vi "Host Main.vi"() -> ()   [LabVIEW 2015]
doc: "This application launches and executes the Tag Bus Data framework configuration for the specified target alias. This is a simple example of the framework API functions, but may also be a suitable starting point for a Host UI or Thick Client that is running a local version of the framework."
uses:
  <vilib>/NI/Module Execution Interface/Engine Runtime/Execution States.ctl
  <vilib>/NI/Module Execution Interface/Engine Runtime/Fault.ctl
  <vilib>/NI/Tag Bus Module Framework/runtime/error classification.ctl
  <vilib>/NI/Module Execution Interface/Engine Runtime/Engine Runtime Interface.lvclass
  <vilib>/NI/DCAF/Tag Editor Core/Framework Configuration Classes/target runtime/PL_Target Runtime.lvclass
  <vilib>/NI/Tag Bus Module Framework/runtime/TBM module execution interface.lvclass
panel:
  in  "configuration file path":path
  in  "target alias":string="PC"
  out "engine status":T4(array[cluster])
  in  "stop":bool
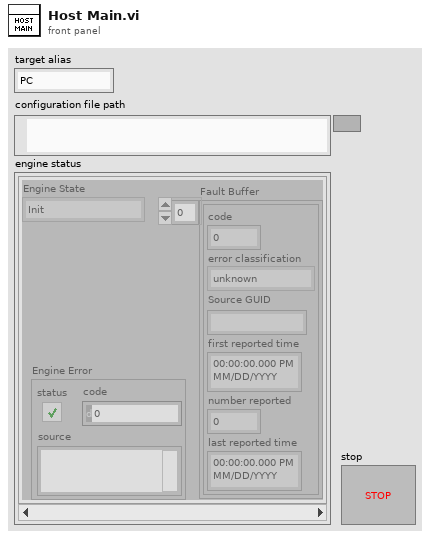
[diagram p1: front panel]
types:
  T1 = typedef "Engine Runtime Interface.lvclass/Execution States.ctl" = enum16{"Init", "Pre-Operational", "Safe-Operational", "Operational", "Stopped"}
  T2 = typedef "Engine Runtime Interface.lvclass/Fault.ctl" = cluster{"code":i32, "error classification":T3, "Source GUID":string, "first reported time":timestamp, "number reported":u32, "last reported time":timestamp}
  T3 = typedef "TBM module execution interface.lvclass/error classification.ctl" = enum16{"unknown", "none", "trivial", "recoverable", "critical"}
  T4 = cluster{"Engine State":T1, "Fault Buffer":T2[], "Engine Error":errorcluster}[]
  T5 = cluster{"Engine State":T1, "Fault Buffer":T2[], "Engine Error":errorcluster}
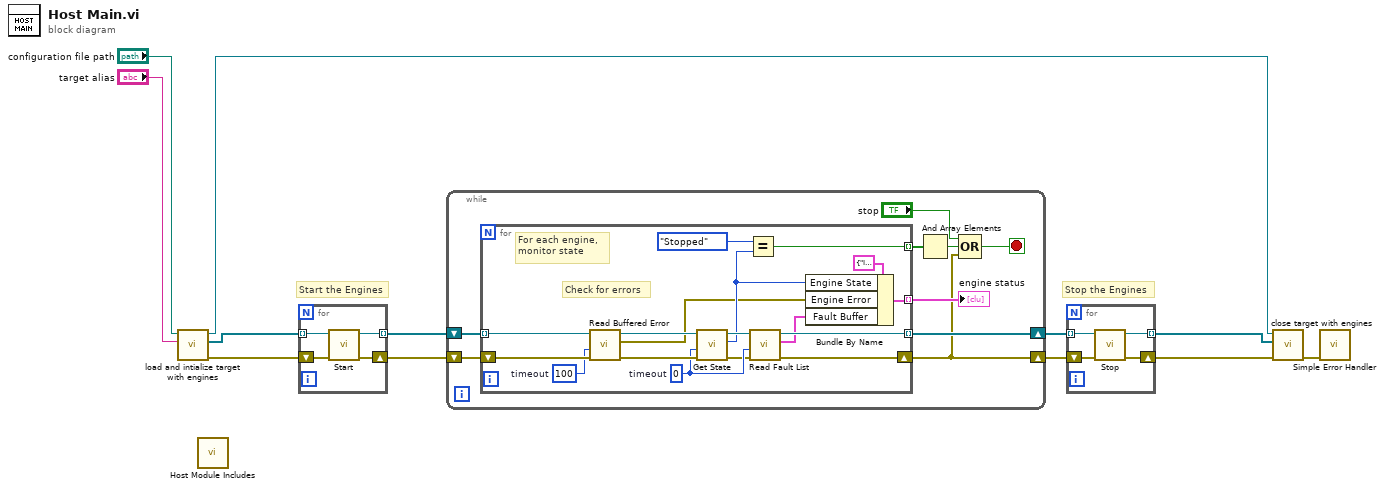
[diagram p0: block diagram]
diagram:
  # "Start the Engines"
  # "Stop the Engines"
  n1 = call <vilib>:"load and intialize target with engines.vi"("target alias"="target alias", "file path"="configuration file path") -> ("error out"=w9:errorcluster, "engine runtime interfaces"=w8:refnum<class "Engine Runtime Interface.lvclass">[], "target runtime"=w5:refnum<class "PL_Target Runtime.lvclass">)  [unwired: 7 in]
  n2 = call "Host Module Includes.vi"() -> ()  [unwired: 12 in]
  n3 = for {
    tunnel: [w16] -> w12 mode=indexing
    tunnel: w8 -> [w13] mode=indexing
    shift-right: [w15] -> w2
    shift-left: w9 -> [w14]
    n4 = call-dynamic "Start.vi"("error in"=w14, "Engine Runtime Interface in"=w13) -> ("error out"=w15:errorcluster, "Engine Runtime Interface out"=w16:refnum<class "Engine Runtime Interface.lvclass">)  [unwired: 8 in]
  }
  n5 = while {
    shift-right: [w23] -> w11
    shift-left: w12 -> [w25]
    shift-right: [w17] -> w10
    shift-left: w2 -> [w24]
    stop <- w21 stop-if-true
    n6 = for {
      tunnel: w25 -> [w42] mode=indexing
      tunnel: [w34] -> w23 mode=indexing
      tunnel: [w37] -> w19 mode=indexing
      shift-right: [w33] -> w17
      shift-left: w24 -> [w41]
      tunnel: [w29] -> w20 mode=indexing
      w32 = 0  # timeout
      w36 = 100  # timeout
      # "For each engine, \nmonitor state"
      # "Check for errors"
      n7 = call-dynamic "Read Buffered Error.vi"("error in"=w41, "timeout in ms (0)"=w36, "Engine Runtime Interface in"=w42) -> ("error out"=w39:errorcluster, "Engine Error"=w27:errorcluster, "Engine Runtime Interface out"=w40:refnum<class "Engine Runtime Interface.lvclass">)  [unwired: 6 in]
      n8 = call-dynamic "Get State.vi"("error in"=w39, "timeout (-1)"=w32, "Engine Runtime Interface in"=w40) -> ("error out"=w26:errorcluster, "Engine State"=w31:T1, "Engine Runtime Interface out"=w35:refnum<class "Engine Runtime Interface.lvclass">)  [unwired: 6 in]
      n9 = Equal?(x=Execution_States."Stopped" ("Engine State"), y=w31) -> (x = y?=w37:bool)
      n10 = call-dynamic "Read Fault List.vi"("error in"=w26, "timeout (-1)"=w32, "Engine Runtime Interface in"=w35) -> ("error out"=w33:errorcluster, "faults"=w30:T2[], "Engine Runtime Interface out"=w34:refnum<class "Engine Runtime Interface.lvclass">)  [unwired: 6 in]
      n11 = Bundle By Name(cluster=T5 {"Engine State"=enum."Init", "Fault Buffer"=[], "Engine Error"={"status"=FALSE, "code"=0, "source"=""}}, "Engine State"=w31, "Engine Error"=w27, "Fault Buffer"=w30) -> (w29:T5)
    }
    "engine status" <- w20
    n12 = And Array Elements(Boolean array=w19) -> (logical AND=w18:bool)
    n13 = Compound Arithmetic op=OR("stop", w18, w17) -> (w21:bool)
  }
  n14 = for {
    tunnel: w11 -> [w46] mode=indexing
    shift-right: [w43] -> w4
    shift-left: w10 -> [w45]
    tunnel: [w44] -> w6 mode=indexing
    n15 = call-dynamic "Stop.vi"("error in"=w45, "Engine Runtime Interface in"=w46) -> ("error out"=w43:errorcluster, "Engine Runtime Interface out"=w44:refnum<class "Engine Runtime Interface.lvclass">)  [unwired: 8 in]
  }
  n16 = call <vilib>:"close target with engines.vi"("error in"=w4, "Engine Runtime Interfaces"=w6, "Target Runtime"=w5) -> ("error out"=w1:errorcluster)  [unwired: 8 in]
  n17 = call <vilib>:"Simple Error Handler.vi"("error in (no error)"=w1) -> ()  [unwired: 4 in, 5 out]
